vi "Read Velocity.vi"(8 "error in (no error)":errorcluster, 11 "PhysicsComponent in":refnum<class "PhysicsComponent.lvclass">) -> (0 "error out":errorcluster, 2 "Velocity out":refnum<class "Vector2.lvclass">, 3 "PhysicsComponent out":refnum<class "PhysicsComponent.lvclass">)   [LabVIEW 2022 SP3, in "PhysicsComponent.lvclass"]
uses:
  PhysicsComponent.lvclass
  Math/Vector2/Vector2.lvclass
  PhysicsComponent.lvclass/PhysicsComponent.ctl
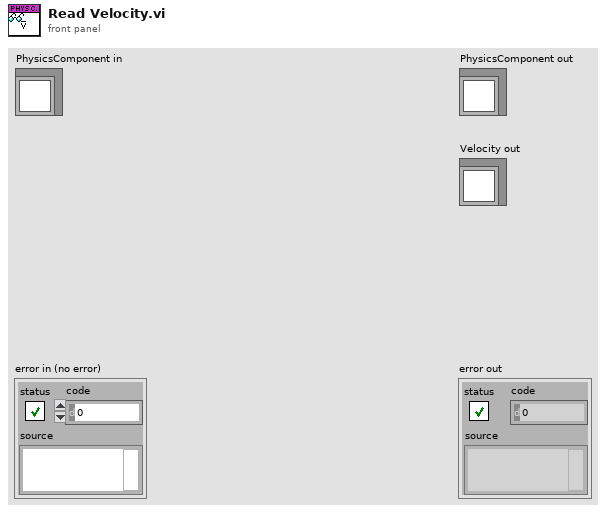
[diagram p1: front panel]
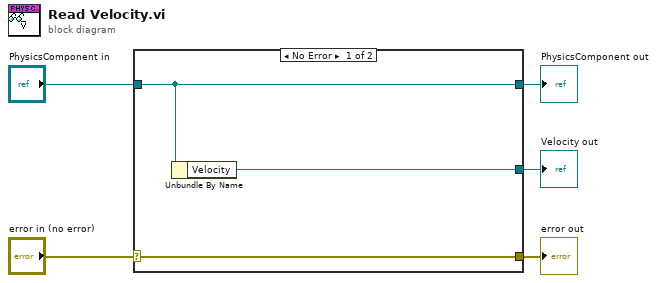
[diagram p0: block diagram]
diagram:
  n1 = case shown="No Error" "error in (no error)" {
    selector: "error in (no error)" -> [w8 w9]
    tunnel: [w8 w9] -> w4
    tunnel: [w7 w10] -> w2
    tunnel: "PhysicsComponent in" -> [w7 w10]
    tunnel: [w6 _] -> w1
    frame No Error {
      n2 = Unbundle By Name(w7) -> ("Velocity"=w6:refnum<class "Vector2.lvclass">)
    }
    frame Error {
    }
  }
  "error out" <- w4
  "PhysicsComponent out" <- w2
  "Velocity out" <- w1
